vi "Misc.vi"() -> ()   [LabVIEW 2018]
uses:
  <vilib>/Rock Robotics/WPI/DriverStation/WPI_DriverStationRobotMode2.ctl
  <vilib>/Rock Robotics/Network Tables/NT Read Boolean.vi
  SubSystems/Drive Train/Drive Train Global.vi
  <vilib>/Rock Robotics/Network Tables/NT Read String.vi
  Robot Global Data.vi
  <vilib>/Rock Robotics/Network Tables/NT Write Number.vi
  SubSystems/HAB Climber/HAB Climber Global.vi
  <vilib>/Rock Robotics/Network Tables/NT Write Boolean.vi
  SubSystems/Lift/Lift Global.vi
  SubSystems/Cargo Intake/Cargo Intake Global.vi
  SubSystems/Hatch Panel Intake/Hatch Panel Intake Global.vi
  <vilib>/Rock Robotics/Network Tables/NT Write Numeric Array.vi
  SubSystems/Controllers/Driver Controller/Driver Controller Global.vi
  SubSystems/Controllers/Manipulator Controlller/Manipulator Controller Global.vi
panel:
  in  "Boolean":bool=TRUE
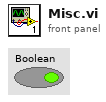
[diagram p1: front panel]
types:
  T1 = typedef "WPI_DriverStationRobotMode2.ctl" = enum16{"Autonomous Disabled", "Autonomous Enabled", "Teleop Disabled", "Teleop Enabled", "Disconnected", "Finish", "Test Disabled", "Test Enabled", "Emergency Stopped"}
  T2 = typedef "WPI_CompressorDevRef.ctl" = cluster{"DevStatus":errorcluster, "Pneumatics Control Module":u8}
  T3 = cluster{"Rollover":dbl, "Yaw":dbl, "Cont Yaw":dbl}
  T4 = cluster{"FrontLeft":dbl, "FrontRight":dbl, "BackLeft":dbl, "BackRight":dbl}
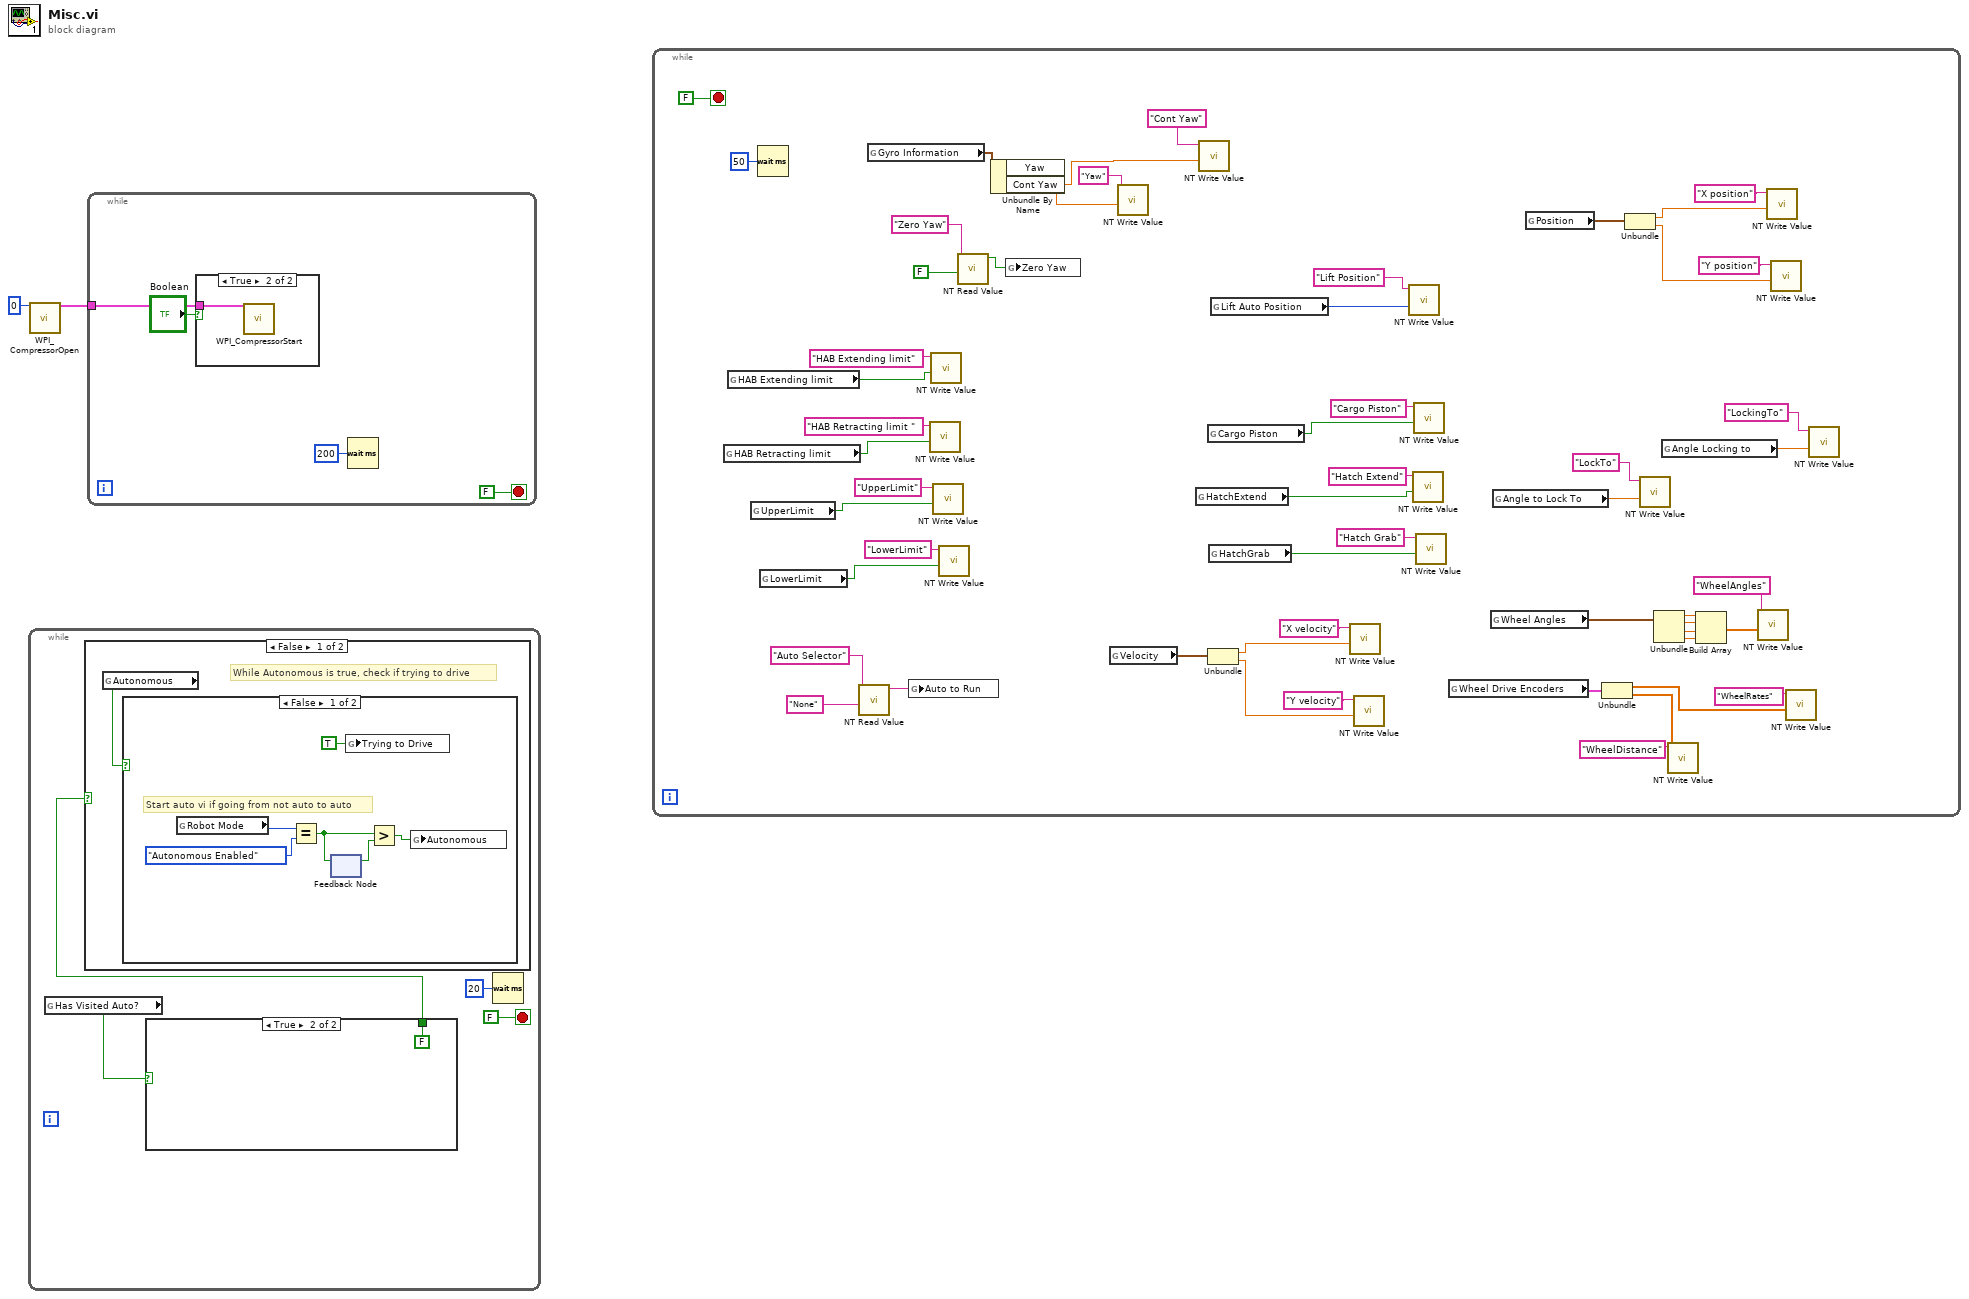
[diagram p0: block diagram]
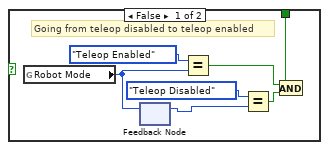
[diagram p2: hidden frame]
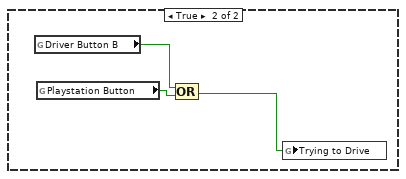
[diagram p3: hidden frame]
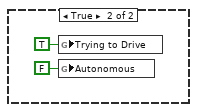
[diagram p4: hidden frame]
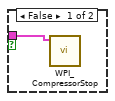
[diagram p5: hidden frame]
diagram:
  n1 = while {
    stop <- FALSE stop-if-true
    n2 = global read "Robot Global Data.vi" "Has Visited Auto?"() -> (w3:bool)
    n3 = case shown="True" w3 {
      tunnel: [w7 FALSE] -> w4
      frame False {
        # "Going from teleop disabled to teleop enabled"
        n4 = global read "Robot Global Data.vi" "Robot Mode"() -> (w13:T1)
        n5 = feedback #1() -> (w10:T1)  [unwired: 1 in]
        n6 = feedback-in #1(w13) -> ()
        n7 = Equal?(x=WPI_DriverStationRobotMode2."Teleop Enabled" ("y"), y=w13) -> (x = y?=w8:bool)
        n8 = Equal?(x=WPI_DriverStationRobotMode2."Teleop Disabled" ("y"), y=w10) -> (x = y?=w9:bool)
        n9 = And(x=w8, y=w9) -> (x .and. y?=w7:bool)
      }
      frame True {
      }
    }
    n10 = case shown="False" w4 {
      frame False {
        # "While Autonomous is true, check if trying to drive"
        n11 = global read "Robot Global Data.vi" "Autonomous"() -> (w15:bool)
        n12 = case shown="False" w15 {
          frame False {
            # "Start auto vi if going from not auto to auto"
            n13 = global read "Robot Global Data.vi" "Robot Mode"() -> (w17:T1)
            n14 = Equal?(x=w17, y=WPI_DriverStationRobotMode2."Autonomous Enabled") -> (x = y?=w18:bool)
            n15 = feedback #2() -> (w19:bool)  [unwired: 1 in]
            n16 = feedback-in #2(w18) -> ()
            n17 = global write "Robot Global Data.vi" "Trying to Drive"(TRUE ("Trying to Drive")) -> ()
            n18 = Greater?(x=w18, y=w19) -> (0:w20:bool)
            n19 = global write "Robot Global Data.vi" "Autonomous"(w20) -> ()
          }
          frame True {
            n20 = global read "Driver Controller Global.vi" "Driver Button B"() -> (w23:bool)
            n21 = global read "Manipulator Controller Global.vi" "Playstation Button"() -> (w22:bool)
            n22 = Compound Arithmetic op=OR(w23, w22) -> (w24:bool)
            n23 = global write "Robot Global Data.vi" "Trying to Drive"(w24) -> ()
          }
        }
      }
      frame True {
        n24 = global write "Robot Global Data.vi" "Trying to Drive"(TRUE ("Trying to Drive")) -> ()
        n25 = global write "Robot Global Data.vi" "Autonomous"(FALSE ("Autonomous")) -> ()
      }
    }
    n26 = Wait (ms)(milliseconds to wait=u32 20) -> ()  [unwired: 1 out]
  }
  n27 = call <vilib>:"WPI_CompressorOpen.vi"("Pneumatics Control Module (0)"=u8 0) -> ("CompressorDevRef"=w1:T2)  [unwired: 13 in, 1 out]
  n28 = while {
    tunnel: w1 -> [w29]
    stop <- FALSE stop-if-true
    n29 = case shown="True" "Boolean" {
      tunnel: w29 -> [w31 w32]
      frame False {
        n30 = call <vilib>:"WPI_CompressorStop.vi"("CompressorDevRef"=w31) -> ()  [unwired: 9 in, 2 out]
      }
      frame True {
        n31 = call <vilib>:"WPI_CompressorStart.vi"("CompressorDevRef"=w32) -> ()  [unwired: 9 in, 2 out]
      }
    }
    n32 = Wait (ms)(milliseconds to wait=u32 200) -> ()  [unwired: 1 out]
  }
  n33 = while {
    stop <- FALSE stop-if-true
    n34 = global read "HAB Climber Global.vi" "HAB Retracting limit"() -> (w73:bool)
    n35 = global read "HAB Climber Global.vi" "HAB Extending limit"() -> (w74:bool)
    n36 = global read "Lift Global.vi" "UpperLimit"() -> (w72:bool)
    n37 = Wait (ms)(milliseconds to wait=u32 50) -> ()  [unwired: 1 out]
    n38 = global read "Lift Global.vi" "LowerLimit"() -> (w71:bool)
    n39 = call-poly <vilib>:"NT Read Value.vi"("Default Value"="None", "Name"="Auto Selector") -> ("String"=w33:string)  [unwired: 8 in, 1 out]
    n40 = global read "Drive Train Global.vi" "Gyro Information"() -> (w81:T3)
    n41 = global write "Robot Global Data.vi" "Auto to Run"(w33) -> ()
    n42 = call-poly <vilib>:"NT Write Value.vi"("Boolean"=w73, "Name"="HAB Retracting limit ") -> ()  [unwired: 9 in, 1 out]
    n43 = call-poly <vilib>:"NT Write Value.vi"("Boolean"=w74, "Name"="HAB Extending limit") -> ()  [unwired: 9 in, 1 out]
    n44 = call-poly <vilib>:"NT Write Value.vi"("Boolean"=w72, "Name"="UpperLimit") -> ()  [unwired: 9 in, 1 out]
    n45 = call-poly <vilib>:"NT Write Value.vi"("Boolean"=w71, "Name"="LowerLimit") -> ()  [unwired: 9 in, 1 out]
    n46 = call-poly <vilib>:"NT Read Value.vi"("Default Value"=FALSE, "Name"="Zero Yaw") -> ("Boolean"=w82:bool)  [unwired: 8 in, 1 out]
    n47 = Unbundle By Name(w81) -> ("Yaw"=w80:dbl, "Cont Yaw"=w79:dbl)
    n48 = global write "Drive Train Global.vi" "Zero Yaw"(w82) -> ()
    n49 = global read "Drive Train Global.vi" "Velocity"() -> (w61:cluster{"X":dbl, "Y":dbl})
    n50 = call-poly <vilib>:"NT Write Value.vi"("Numeric"=w80, "Name"="Yaw") -> ()  [unwired: 9 in, 1 out]
    n51 = global read "Hatch Panel Intake Global.vi" "HatchExtend"() -> (w65:bool)
    n52 = call-poly <vilib>:"NT Write Value.vi"("Numeric"=w79, "Name"="Cont Yaw") -> ()  [unwired: 9 in, 1 out]
    n53 = global read "Cargo Intake Global.vi" "Cargo Piston"() -> (w66:bool)
    n54 = Unbundle(w61) -> ("X"=w59:dbl, "Y"=w57:dbl)
    n55 = global read "Hatch Panel Intake Global.vi" "HatchGrab"() -> (w64:bool)
    n56 = global read "Lift Global.vi" "Lift Auto Position"() -> (w62:u16)
    n57 = call-poly <vilib>:"NT Write Value.vi"("Numeric"=w59, "Name"="X velocity") -> ()  [unwired: 9 in, 1 out]
    n58 = call-poly <vilib>:"NT Write Value.vi"("Numeric"=w57, "Name"="Y velocity") -> ()  [unwired: 9 in, 1 out]
    n59 = call-poly <vilib>:"NT Write Value.vi"("Numeric"=w62, "Name"="Lift Position") -> ()  [unwired: 9 in, 1 out]
    n60 = call-poly <vilib>:"NT Write Value.vi"("Boolean"=w65, "Name"="Hatch Extend") -> ()  [unwired: 9 in, 1 out]
    n61 = call-poly <vilib>:"NT Write Value.vi"("Boolean"=w66, "Name"="Cargo Piston") -> ()  [unwired: 9 in, 1 out]
    n62 = call-poly <vilib>:"NT Write Value.vi"("Boolean"=w64, "Name"="Hatch Grab") -> ()  [unwired: 9 in, 1 out]
    n63 = global read "Drive Train Global.vi" "Wheel Drive Encoders"() -> (w49:cluster{"Rates":dbl[], "Distances":dbl[]})
    n64 = global read "Drive Train Global.vi" "Wheel Angles"() -> (w56:T4)
    n65 = global read "Drive Train Global.vi" "Angle to Lock To"() -> (w43:dbl)
    n66 = global read "Drive Train Global.vi" "Position"() -> (w36:cluster{"X":dbl, "Y":dbl})
    n67 = Unbundle(w49) -> ("Rates"=w45:dbl[], "Distances"=w48:dbl[])
    n68 = Unbundle(w36) -> ("X"=w38:dbl, "Y"=w40:dbl)
    n69 = call-poly <vilib>:"NT Write Value.vi"("Numeric"=w43, "Name"="LockTo") -> ()  [unwired: 9 in, 1 out]
    n70 = Unbundle(w56) -> ("FrontLeft"=w52:dbl, "FrontRight"=w53:dbl, "BackLeft"=w54:dbl, "BackRight"=w55:dbl)
    n71 = global read "Drive Train Global.vi" "Angle Locking to"() -> (w42:dbl)
    n72 = call-poly <vilib>:"NT Write Value.vi"("Numeric Array"=w48, "Name"="WheelDistance") -> ()  [unwired: 9 in, 1 out]
    n73 = Build Array(w52, w53, w54, w55) -> (w51:dbl[])
    n74 = call-poly <vilib>:"NT Write Value.vi"("Numeric Array"=w51, "Name"="WheelAngles") -> ()  [unwired: 9 in, 1 out]
    n75 = call-poly <vilib>:"NT Write Value.vi"("Numeric"=w38, "Name"="X position") -> ()  [unwired: 9 in, 1 out]
    n76 = call-poly <vilib>:"NT Write Value.vi"("Numeric"=w40, "Name"="Y position") -> ()  [unwired: 9 in, 1 out]
    n77 = call-poly <vilib>:"NT Write Value.vi"("Numeric Array"=w45, "Name"="WheelRates") -> ()  [unwired: 9 in, 1 out]
    n78 = call-poly <vilib>:"NT Write Value.vi"("Numeric"=w42, "Name"="LockingTo") -> ()  [unwired: 9 in, 1 out]
  }
